vi "_main.vi"() -> ()   [LabVIEW 2012]
panel:
  in  "milliseconds to wait":u32=1000
  in  "stop":bool
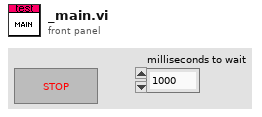
[diagram p1: front panel]
types:
  T1 = typedef "LabVIEWHTTPClient.lvlib/ClientHandle.ctl" = refnum<k1>
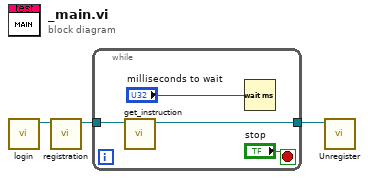
[diagram p0: block diagram]
diagram:
  n1 = call "login.vi"() -> ("client handle out"=w3:T1)  [unwired: 11 in]
  n2 = call "registration.vi"("client handle"=w3) -> ("client handle out"=w2:T1)  [unwired: 10 in]
  n3 = while {
    tunnel: w2 -> [w7]
    tunnel: [w4] -> w1
    stop <- "stop" stop-if-true
    n4 = call "get_instruction.vi"("client handle"=w7) -> ("client handle out"=w4:T1)  [unwired: 10 in]
    n5 = Wait (ms)(milliseconds to wait="milliseconds to wait") -> ()  [unwired: 1 out]
  }
  n6 = call "Unregister.vi"("client handle"=w1) -> ()  [unwired: 11 in]
